vi "calc Ramp Time.vi"(0 "Stop":dbl, 1 "Start":dbl, 2 "Dwell (ms)":dbl, 3 "Scan Type":u8, 4 "Step":dbl) -> (5 "Ramp Time (ms)":i32)   [LabVIEW 2018]
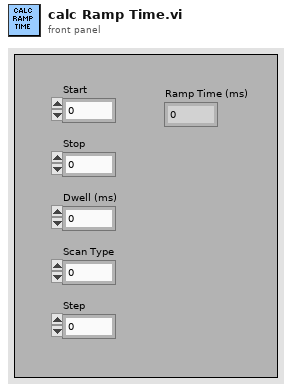
[diagram p1: front panel]
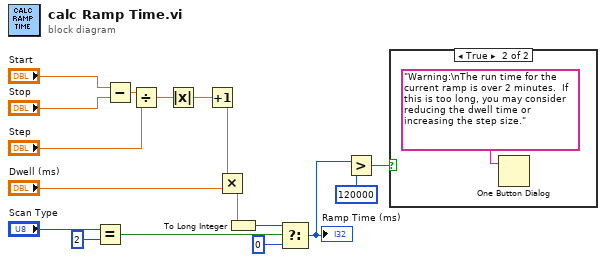
[diagram p0: block diagram]
diagram:
  n1 = Equal?(x="Scan Type", y=u8 2) -> (x = y?=w10:bool)
  n2 = Subtract(x="Start", y="Stop") -> (x-y=w7:dbl)
  n3 = Divide(x=w7, y="Step") -> (x/y=w6:dbl)
  n4 = Absolute Value(x=w6) -> (abs(x)=w5:dbl)
  n5 = Increment(x=w5) -> (x+1=w14:dbl)
  n6 = Multiply(x=w14, y="Dwell (ms)") -> (x*y=w16:dbl)
  n7 = To Long Integer(number=w16) -> (32bit integer=w4:i32)
  n8 = Select(t=w4, s=w10, f=0) -> (s? t:f=w3:i32)
  "Ramp Time (ms)" <- w3
  n9 = Greater?(x=w3, y=120000) -> (0:w1:bool)
  n10 = case shown="True" w1 {
    frame False {
    }
    frame True {
      n11 = One Button Dialog(message="Warning:\nThe run time for the current ramp is over 2 minutes.  If this is too long, you may consider reducing the dwell time or increasing the step size.") -> ()  [unwired: 2 out]
    }
  }
